vi "Low-Level Stream to Text File (NChan NSamp).vi"() -> ()   [LabVIEW 2020]
uses:
  <vilib>/DAQmx/read.llb/DAQmx Read (Analog 2D DBL NChan NSamp).vi
  <vilib>/DAQmx/create/channels.llb/DAQmx Create Channel (AI-Voltage-Basic).vi
  <vilib>/DAQmx/configure/timing.llb/DAQmx Timing (Sample Clock).vi
  <vilib>/DAQmx/miscellaneous.llb/DAQmx Fill In Error Info.vi
  <resource>/objmgr/daqmx.rc
panel:
  in  "stop":bool
  out "Waveform Chart":dbl[][](graph)
  in  "minimum value":dbl=-5.0
  in  "maximum value":dbl=5.0
  in  "Number of Samples":i32=5
  in  "Desired Sample Rate (Hz)":dbl=10.0
  in  "Physical Channels":tag="PCI-6221/ai0:3"
  out "Actual Sample Rate (Hz)":dbl
  # "Measurement Range"
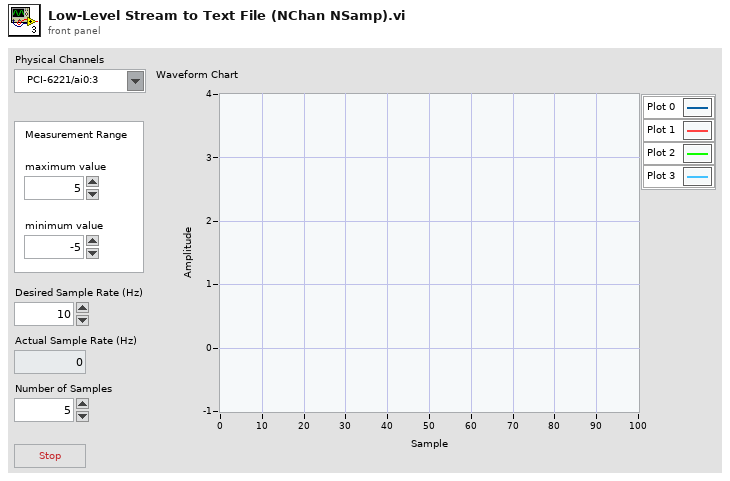
[diagram p1: front panel]
types:
  T1 = enum16{"open", "replace", "create", "open or create", "replace or create", "replace or create with confirmation"}
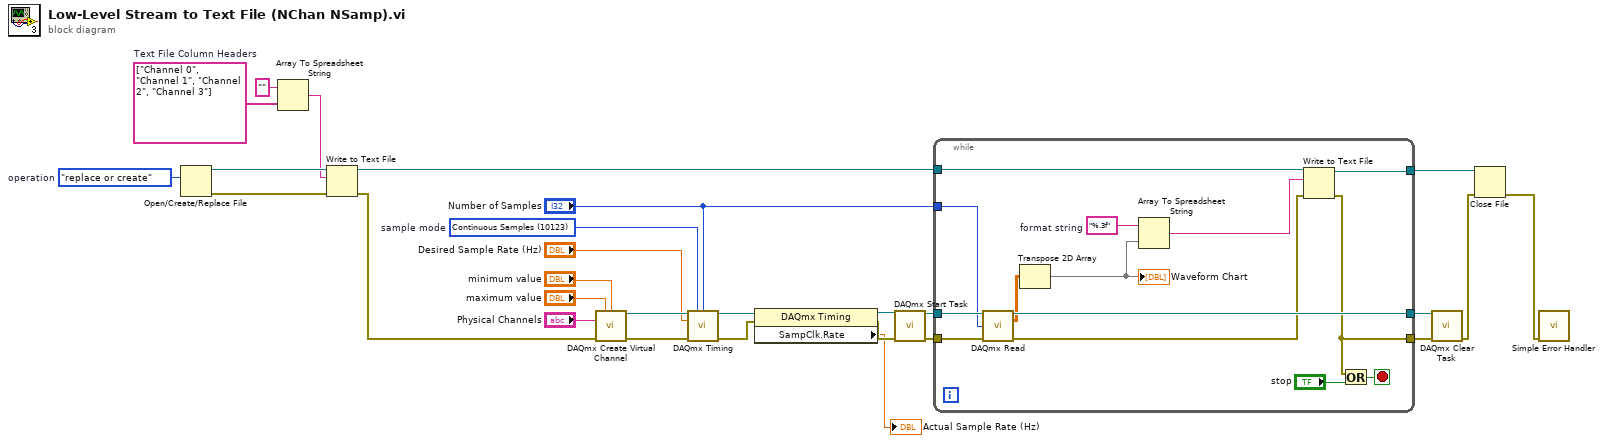
[diagram p0: block diagram]
diagram:
  w13 = string[] ["Channel 0", "Channel 1", "Channel 2", "Channel 3"]  # Text File Column Headers
  w17 = T1."replace or create"  # operation
  w24 = 10123 items=["Finite Samples"=10178, "Continuous Samples"=10123, "Hardware Timed Single Point"=12522]  # sample mode
  n1 = Open/Create/Replace File(operation (0:open)=w17) -> (refnum out=w19:refnum<file>, error out=w18:errorcluster)  [unwired: 5 in, 1 out]
  n2 = Array To Spreadsheet String(array=w13, 3:"") -> (spreadsheet string=w12:string)  [unwired: 1 in]
  n3 = Write to Text File(file (use dialog)=w19, text=w12, error in=w18) -> (refnum out=w20:refnum<file>, error out=w21:errorcluster)  [unwired: 1 in, 1 out]
  n4 = call-poly <vilib>:"DAQmx Create Virtual Channel.vi"("maximum value"="maximum value", "minimum value"="minimum value", "physical channels"="Physical Channels", "error in"=w21) -> ("task out"=w28:refnum<k21>, "error out"=w27:errorcluster)  [unwired: 10 in]
  n5 = call-poly <vilib>:"DAQmx Timing.vi"("task/channels in"=w28, "sample mode"=w24, "samples per channel"="Number of Samples", "rate"="Desired Sample Rate (Hz)", "error in"=w27) -> ("task out"=w10:refnum<k21>, "error out"=w9:errorcluster)  [unwired: 9 in]
  n6 = property class="DAQmx Timing"(reference=w10, error in=w9) -> (reference out=w8:refnum<k21>, error out=w7:errorcluster, "SampClk.Rate"=→"Actual Sample Rate (Hz)":dbl)
  n7 = call <vilib>:"DAQmx Start Task.vi"("task/channels in"=w8, "error in"=w7) -> ("task out"=w26:refnum<k21>, "error out"=w25:errorcluster)  [unwired: 12 in]
  n8 = while {
    tunnel: w26 -> [w42]
    tunnel: w25 -> [w41]
    tunnel: [w40] -> w23
    tunnel: [w36] -> w22
    tunnel: w20 -> [w38]
    tunnel: [w37] -> w16
    tunnel: "Number of Samples" -> [w32]
    stop <- w39 stop-if-true
    w35 = "%.3f"  # format string
    n9 = call-poly <vilib>:"DAQmx Read.vi"("task/channels in"=w42, "number of samples per channel"=w32, "error in"=w41) -> ("task out"=w40:refnum<k21>, "data"=w31:dbl[][], "error out"=w33:errorcluster)  [unwired: 10 in]
    n10 = Transpose 2D Array(2D array=w31) -> (transposed array=w30:dbl[][])
    "Waveform Chart" <- w30
    n11 = Array To Spreadsheet String(array=w30, 3:w35) -> (spreadsheet string=w34:string)  [unwired: 1 in]
    n12 = Write to Text File(file (use dialog)=w38, text=w34, error in=w33) -> (refnum out=w37:refnum<file>, error out=w36:errorcluster)  [unwired: 1 in, 1 out]
    n13 = Or(x=w36, y="stop") -> (x .or. y?=w39:bool)
  }
  n14 = call <vilib>:"DAQmx Clear Task.vi"("task in"=w23, "error in"=w22) -> ("error out"=w15:errorcluster)  [unwired: 13 in]
  n15 = Close File(refnum=w16, error in=w15) -> (error out=w14:errorcluster)  [unwired: 1 out]
  n16 = call <vilib>:"Simple Error Handler.vi"("error in (no error)"=w14) -> ()  [unwired: 4 in, 5 out]
